vi "ni579x Configure Clock Phase DAC.vi"(0 "Register Bus":T1, 1 "scope":string(combo), 5 "clock phase DAC value":u16=32768, 11 "Error In":errorcluster) -> (4 "Register Bus (out)":T1, 6 "coerced clock phase DAC value":u16, 15 "Error Out":errorcluster)   [LabVIEW 2015, in "ni579x Config v2 Host.lvlib"]
doc: "Configures the value of the clock phase DAC. Modifies the phase of the reference used to generate the sample clock and LO if the reference frequency source is external.\n\n<B>Input Parameters</B>\n\n<B>Register Bus</B> The Register Bus object created by the ni579x Open VI and used as the session handle for the NI-579x Configuration Design Library.\n\n<B>scope</B> Ignored.\n\n<B>clock phase DAC value</B> The value to set to the clock phase DAC.\n\n<B>Output Parameters</B>\n\n<B>Register Bus (out)</B> The Register Bus object created by the ni579x Open VI and used as the session handle for the NI-579x Configuration Design Library.\n\n<B>coerced clock phase DAC value</B> The coerced value programmed to the clock phase DAC."
uses:
  <instrlib>/ni579x/Config/v2/Host/ni579x Config v2 Host.lvlib
  <instrlib>/_niInstr/Register Bus/v0/Host/Public/Register Bus Session.ctl
  <instrlib>/_niInstr/Register Bus/v0/Host/Private/Session Data.ctl
  <instrlib>/_niInstr/Register Bus/v0/Host/niInstr Register Bus v0 Host.lvlib
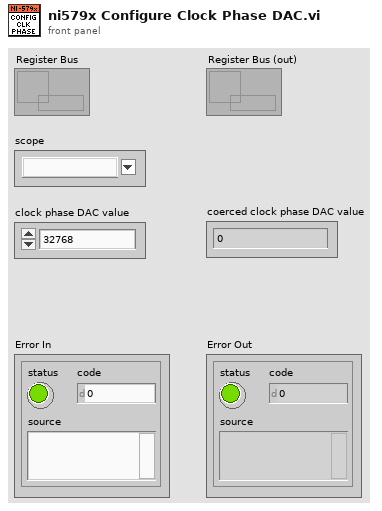
[diagram p1: front panel]
types:
  T1 = typedef "niInstr Register Bus v0 Host.lvlib/Register Bus Session.ctl" = refnum<queue>
  T2 = typedef "ni579x Config v2 Shared.lvlib/ni579x FAM Register Operation.ctl" = cluster{"FAM Register Offset":T3, "Address":u32, "Write (T)/Read (F)":bool, "Write Data":u32}
  T3 = typedef "ni579x Config v2 Shared.lvlib/ni579x FAM Register Offset.ctl" = u8
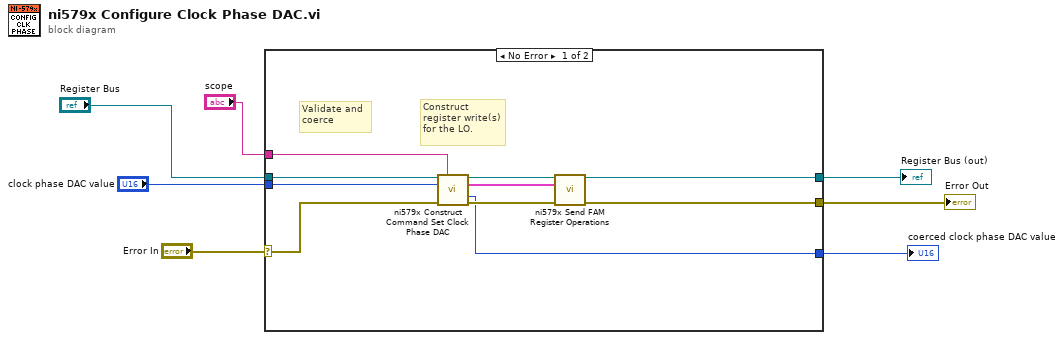
[diagram p0: block diagram]
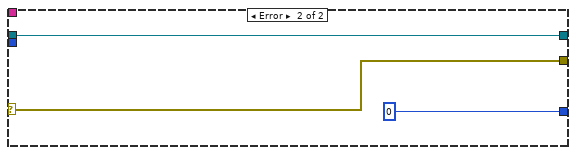
[diagram p2: hidden frame]
diagram:
  n1 = case shown="No Error" "Error In" {
    selector: "Error In" -> [w8 w20]
    tunnel: [w13 w20] -> w6
    tunnel: "Register Bus" -> [w9 w19]
    tunnel: "clock phase DAC value" -> [w10 _]
    tunnel: [w14 w19] -> w3
    tunnel: [w11 u16 0 ("coerced attenuation [dB]")] -> w2
    tunnel: "scope" -> [w12 _]
    frame No Error {
      # "Construct\nregister write(s)\nfor the LO."
      # "Validate and \ncoerce"
      n2 = call <instrlib>:"ni579x Construct Command Set Clock Phase DAC.vi"("Register Bus"=w9, "scope"=w12, "clock phase DAC value"=w10, "Error In"=w8) -> ("Register Bus (out)"=w17:T1, "FAM Register Operations"=w15:T2[], "coerced clock phase DAC value"=w11:u16, "Error Out"=w16:errorcluster)  [unwired: 8 in]
      n3 = call <instrlib>:"ni579x Send FAM Register Operations.vi"("Register Bus"=w17, "FAM Register Operations"=w15, "Error In"=w16) -> ("Register Bus (out)"=w14:T1, "Error Out"=w13:errorcluster)  [unwired: 10 in, 1 out]
    }
    frame Error {
    }
  }
  "Register Bus (out)" <- w3
  "Error Out" <- w6
  "coerced clock phase DAC value" <- w2
